vi "Dashboard Main.vi"() -> ()   [LabVIEW 2015]
uses:
  <vilib>/Utility/miscctls.llb/LVRowAndColumnTypeDef.ctl
  <vilib>/event_ctls.llb/eventvkey.ctl
  <vilib>/Rock Robotics/WPI/Dashboard/WPI_DashboardLogging Global.vi
  <vilib>/picture/3D Picture Control/Object/Create Object (name).vi
  <vilib>/Rock Robotics/Network Tables/NT Read Numeric Array.vi
  <vilib>/Rock Robotics/Network Tables/NT Write Boolean.vi
  <vilib>/Rock Robotics/Network Tables/NT Read Boolean Array.vi
  <vilib>/Rock Robotics/Network Tables/NT Read Boolean.vi
  <vilib>/Rock Robotics/Network Tables/NT Write String Array.vi
  <vilib>/Rock Robotics/Network Tables/NT Write Numeric Array.vi
  <vilib>/Utility/config.llb/Write Key (String).vi
  <vilib>/Utility/config.llb/Write Key (I32).vi
  <vilib>/Utility/config.llb/NI_LVConfig.lvlib
  <vilib>/picture/3D Picture Control/NI_3D Picture Control.lvlib
panel:
  out "NT Connected":bool
  in  "TCP":refnum<k5>
  in  "Rec Mode":enum32{"Stop", "Record", "Playback"}(radio)
  in  "Vision":u16(ring) items=["Camera Off", "USB Camera SW", "USB Camera HW", "IP Camera"]
  out "Camera IP":string
  out "Image Message":string="Timeout in Camera Communications"
  in  "Dashboard Tab":T1(tab)
  out "DD Up?":bool
  out "Intake Up?":bool
  out "Gyro Z Angle":dbl format="%#_4f"
  in  "Custom Drive?":bool=TRUE
  in  "Refresh \nRoutines":bool
  in  "Auto Routines":string(combo)
  in  "Camera Settings":T2={"Frame Rate"=30, "Compression"=30, "Size"=1} {"Frame Rate" scale=1.0..30.0; "Size" items=["640x480", "320x240", "160x120"]}
  out "MotorChart R":cluster{"Numeric":dbl, "Numeric":dbl}(graph)
  out "MotorChart L":T3(graph)
  out "MotorSliders R":cluster{"MotorSlide1":dbl, "MotorSlide2":dbl} {"MotorSlide2" scale=-1.0..1.0 scale format="%#_2e"; "MotorSlide1" scale=-1.0..1.0 scale format="%#_2e"}
  out "MotorSliders L":T4 {"MotorSlide4 2" scale=0.0..14.0 scale format="%#_2e"; "MotorSlide2" scale=-1.0..1.0 scale format="%#_2e"; "MotorSlide1" scale=-1.0..1.0 scale format="%#_2e"}
  out "Gyro Z Angle":dbl(knob) scale=0.0..360.0
  out "JS1 Z":dbl(slide) scale=-1.0..1.0 scale format="%#_2e"
  out "JS1 Graph":cluster{"X":dbl, "Y":dbl}[](graph)
  out "JS1 Buttons":T5
  out "JS2 Z":dbl(slide) scale=-1.0..1.0 scale format="%#_2e"
  out "JS2 Graph":cluster{"X":dbl, "Y":dbl}[](graph)
  out "JS2 Buttons":T5
  out "Mode":T6(ring)=enum."Auto Disabled"
  in  "DB Camera Config":bool
  out "fps":dbl format="%#.1g"
  out "Mbps":dbl format="%#.1g"
  out "Mbps 2":bool
  out "Robot Current":T7(graph)
  out "Compressor On?":bool
  out "System Current":T7(graph)
  out "Robot Position":refnum<vi>(3d-picture)
  out "IMU Angle":cluster{"X":dbl, "Y":dbl, "Z":dbl}
  out "IMU AHRS":cluster{"Pitch":dbl, "Roll":dbl, "Yaw":dbl}
  out "Right Encoder":dbl(knob) scale=0.0..256.0
  out "Right Encoder Numeric":dbl
  out "Left Encoder Numeric":dbl
  out "Left Encoder":dbl(knob) scale=0.0..256.0
  out "Tree":string(tree)
  in  "Test Slider":dbl(slide) scale=0.0..100.0 scale format="%#_3g"
  in  "On/Off":bool caption="Solenoid"
  in  "Test Name":u16(ring) items=["Select the test to run..."]
  in  "Test Tree":string(tree)
  in  "Motor":cluster{"Value":dbl, "Enable":bool} {"Value" scale=-1.0..1.0 scale format="%#_3g"}
  out "Progress":T8 {"Test Progress" scale=0.0..100.0}
  in  "Rev/Fwd":cluster{"Forward":bool, "Reverse":bool}
  in  "Test Ring":u16(ring) items=["Monochrome", "Color"]
  out "Cmd Status":string
  in  "Execute Command":bool
  in  "Command Params":string[][](table)
  in  "Command Selection":i32(listbox)
  in  "CheckList":i32(listbox)
  out "Camera Image":T9(plugin-control)
  out "Boolean":bool
  # "Left"
  # "Front"
  # "Right"
  # "Battery"
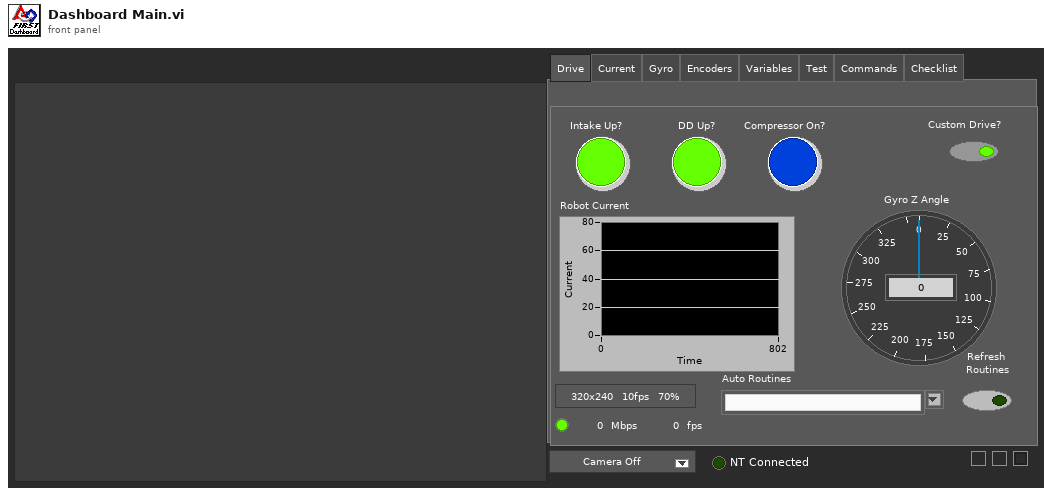
[diagram p1: front panel]
types:
  T1 = enum32{"Drive", "Current", "Gyro", "Encoders", "Variables", "Test", "Commands", "Checklist"}
  T2 = cluster{"Frame Rate":i32, "Compression":i32, "Size":u16}
  T3 = cluster{"Numeric":dbl, "Numeric":dbl, "Battery V":dbl}
  T4 = cluster{"MotorSlide1":dbl, "MotorSlide2":dbl, "MotorSlide4 2":dbl}
  T5 = cluster{bool, bool, bool, bool, bool, bool, bool, bool, bool, bool, bool, bool}
  T6 = enum8{"Tele-Op Disabled", "Tele-Op Enabled", "Auto Disabled", "Auto Enabled", "Test Disabled", "Test Enabled", "Disconnected", "No Code", "E-Stop"}
  T7 = cluster{"Numeric":dbl, "Numeric":dbl, "Numeric":dbl, "Numeric":dbl, "Numeric":dbl}
  T8 = cluster{"Test Progress":u8, "Test Progress Text":string}
  T9 = typedef "IMAQ Image.ctl" = refnum<image>
  T10 = cluster{"IDs":cluster{"RPC field ID":u16, "Unique ID":u16}, "String":string}
  T11 = enum32{"Drive", "Basic", "Custom", "Test", "Checklist", "Variables"}
  T12 = typedef "Image Type" = u32
  T13 = cluster{"Camera Image":refnum<vi>, "Dashboard Tab":refnum<vi>, "Boolean":refnum<vi>, "Vision":refnum<vi>, "Rec Mode":refnum<vi>, "Test Slider":refnum<vi>, "On/Off ":refnum<vi>, "Test Ring":refnum<vi>, "Rev/Fwd":refnum<vi>, "Test Name":refnum<vi>, "Motor":refnum<vi>, "Progress":refnum<vi>, "CheckList":refnum<vi>, "Tree":refnum<vi>, "Test Tree":refnum<vi>, "Command Params":refnum<vi>, "Command Selection":refnum<vi>, "Execute Command":refnum<vi>, "Cmd Status":refnum<vi>}
  T14 = cluster{"Match Time":dbl, "Left Master":dbl, "Left Slave":dbl, "Right Master":dbl, "Right Slave":dbl, "Battery V":dbl, "Pitch":dbl, "Roll":dbl, "Yaw":dbl, "X Angle":dbl, "Y Angle":dbl, "Z Angle":dbl, "Compressor I":dbl}
  T15 = cluster{"Error Strings":string, "Disable Counts":cluster{u16, u16}, "Rail Faults":cluster{u16, u16, u16}, "Robot IP":string, "DB Mode":u8, "Event Info":cluster{"Name":string, "Type":u8, "Number":u16, "Replay":u8}, "Camera Addr":string}
  T16 = cluster{"Storage":cluster{"Disk Free":u64, "RAM Block":u32, "RAM free":u32}, "CPU Utilization":cluster{"CPU % ISR":sgl, "CPU % Time Crit":sgl, "CPU % Timed Str":sgl, "CPU % High":sgl, "CPU % Above":sgl, "CPU % Normal":sgl, "CPU % Low":sgl}, "CAN":cluster{"% Bus Utilization":sgl, "Bus Off Cnt":u32, "TX_FIFO Full Cnt":u32, "Receive Error Cnt":u8, "Transmit Error Cnt":u8}, "HID":cluster{"HID Outputs":u32, "Rumble Low":u16, "Rumble High":u16}[]}
  T17 = cluster{"Status bits":cluster{"Test Mode":bool, "Autonomous":bool, "Enabled":bool, "Code Start":bool, "Brownout":bool, "Reserved 2":bool, "Reserved 3":bool, "E-Stop":bool}, "Code Trace":cluster{"Disabled":bool, "TeleOp":bool, "Auto":bool, "Test":bool}, "Controller Type":enum16{"unknown", "cRIO", "roboRio"}, "Code?":enum16{"unknown", "noCode", "code"}, "Battery V":dbl}
  T18 = cluster{"Control Bits":cluster{"TestMode":bool, "Autonomous":bool, "Enabled":bool, "FMS Present":bool, bool, bool, bool, "E-Stop":bool}, "Team Station ":u8, "Countdown":sgl, "Joystick Values":cluster{"Axes":dbl[], "Buttons":bool[], "POVs":i16[]}[]}
  T19 = cluster{"Axes":dbl[], "Buttons":bool[], "POVs":i16[]}[]
  T20 = cluster{"Numeric Array[0]":dbl, "Numeric Array[1]":dbl, "Numeric Array[2]":dbl, "Numeric Array[3]":dbl, "Numeric Array[4]":dbl, "Numeric Array[5]":dbl, "Numeric Array[6]":dbl, "Numeric Array[7]":dbl, "Numeric Array[8]":dbl}
  T21 = cluster{"Axes":dbl[], "Buttons":bool[], "POVs":i16[]}
  T22 = cluster{"Buttons[0]":bool, "Buttons[1]":bool, "Buttons[2]":bool, "Buttons[3]":bool, "Buttons[4]":bool, "Buttons[5]":bool, "Buttons[6]":bool, "Buttons[7]":bool, "Buttons[8]":bool, "Buttons[9]":bool, "Buttons[10]":bool, "Buttons[11]":bool}
  T23 = typedef "NI_LVConfig.lvlib/Config Data RefNum.ctl" = refnum<k1>
  T24 = cluster{"Operation":enum16{"Update", "Clear"}, "Color Box":u32}[]
  T25 = typedef "eventvkey.ctl" = enum16{"ASCII", "Enter", "Return", "Shift", "Ctrl", "Alt", "Cmd", "Opt", "Caps", "NumLock", "Clear", "Break", "Up", "Down", "Left", "Right", "Insert", "Delete", "Home", "End", "PageUp", "PageDown", "Escape", "Help", "Pause", "ScrollLock", "F1", "F2", "F3", "F4", "F5", "F6", "F7", "F8", "F9", "F10", "F11", "F12", "F13", "F14", "F15", "F16", "F17", "F18", "F19", "F20", "F21", "F22", "F23", "F24", "Play", "VolumeUp", "VolumeDown", "Mute", "Two Byte Char"}
  T26 = cluster{"Image Size":bool, "Image Type":bool, "Pixel Value":bool, "ROI Information":bool, "Zoom Factor":bool}
  T27 = enum8{"Enabled", "Disabled", "Disabled and Grayed Out"}
  T28 = cluster{"Operation":enum16{"Update", "Clear"}, "Color Box":u32}
  T29 = typedef "LVRowAndColumnTypeDef.ctl" = cluster{"Row":i32, "Column":i32}
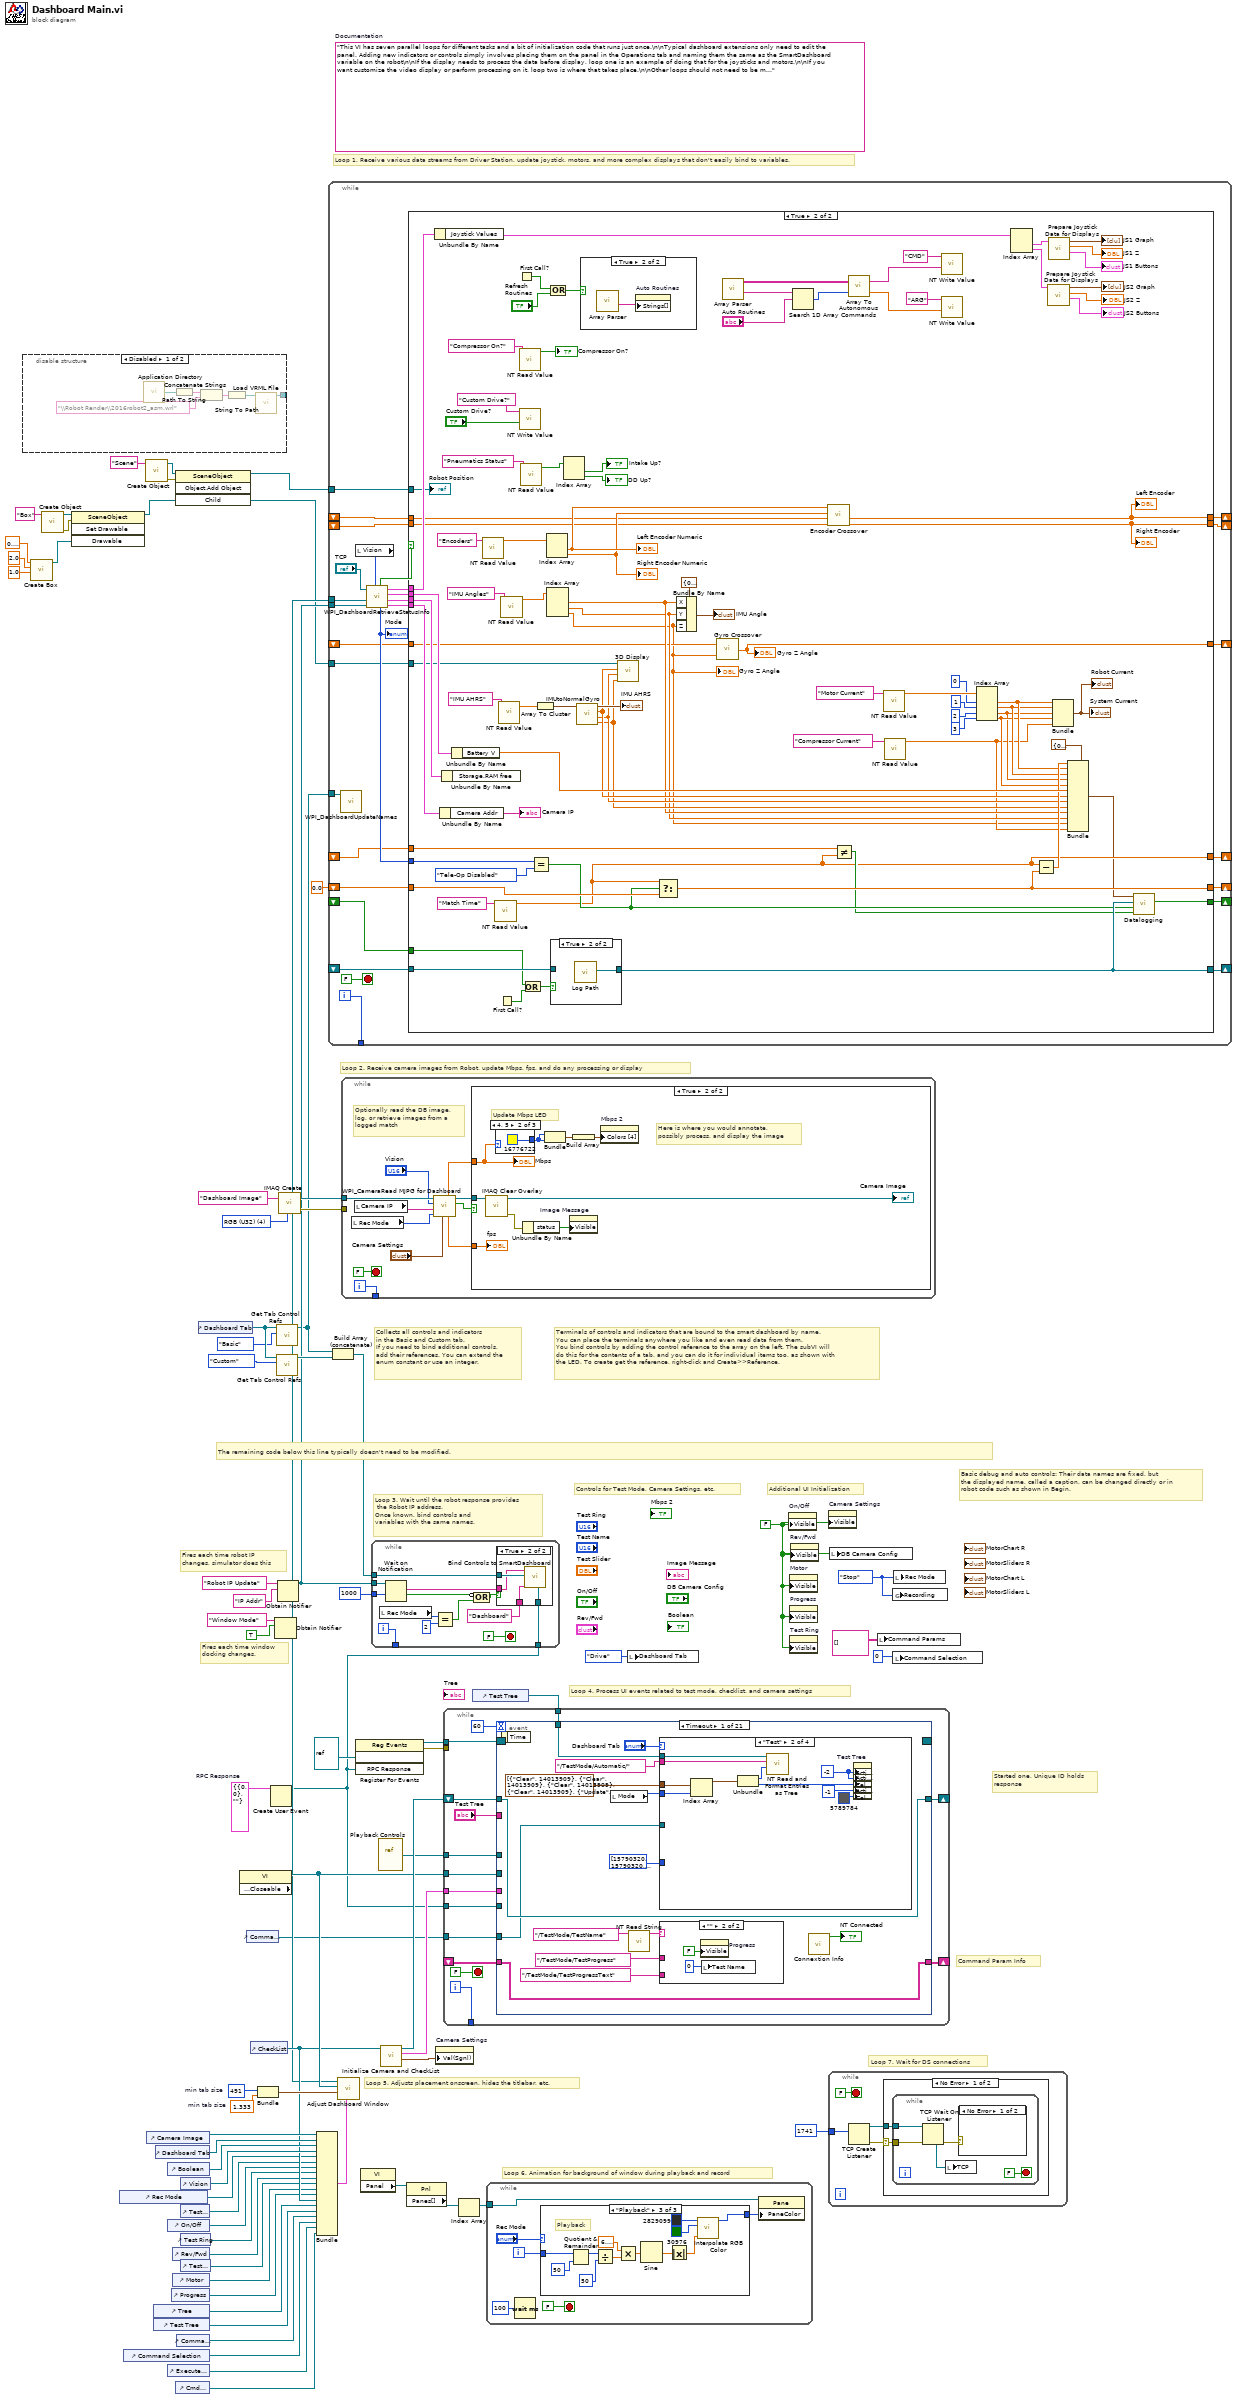
[diagram p0: block diagram]
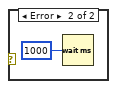
[diagram p3: hidden frame]
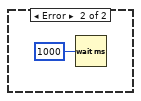
[diagram p4: hidden frame]
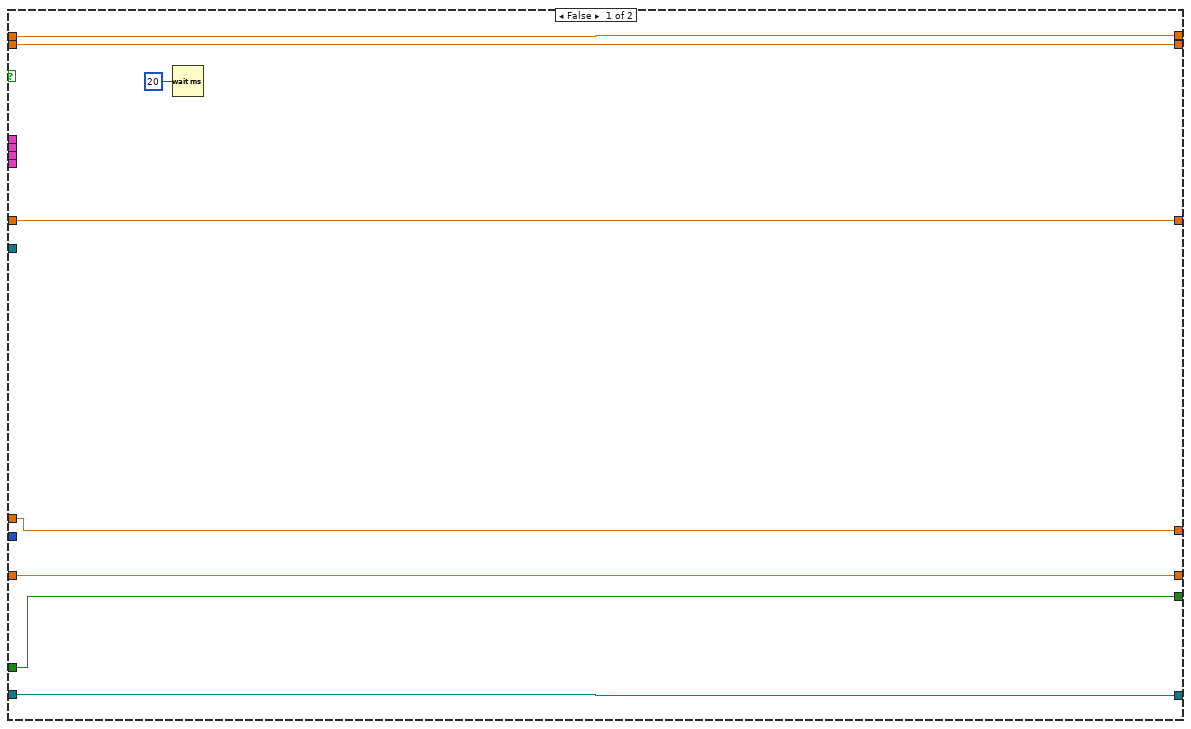
[diagram p5: hidden frame]
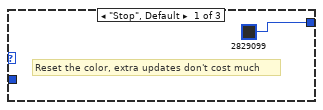
[diagram p8: hidden frame]
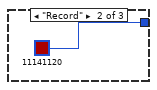
[diagram p9: hidden frame]
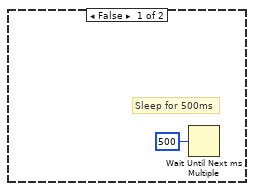
[diagram p11: hidden frame]
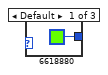
[diagram p12: hidden frame]
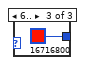
[diagram p13: hidden frame]
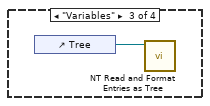
[diagram p15: hidden frame]
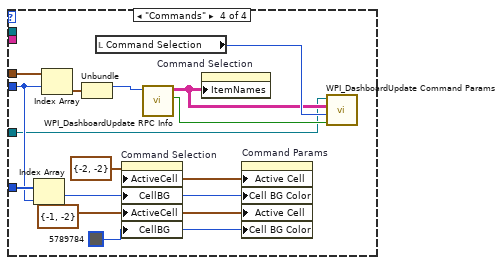
[diagram p16: hidden frame]
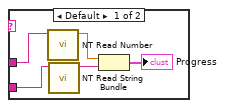
[diagram p17: hidden frame]
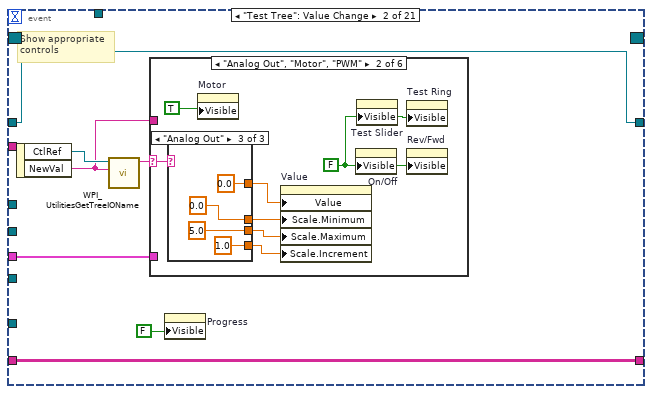
[diagram p18: hidden frame]
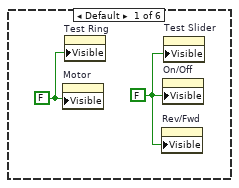
[diagram p19: hidden frame]
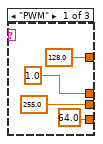
[diagram p20: hidden frame]
diagram:
  w22 = T10 {"IDs"={"RPC field ID"=0, "Unique ID"=0}, "String"=""}  # RPC Response
  w47 = 491  # min tab size
  w46 = 1.333  # min tab size
  w55 = enum32{"Stop", "Record", "Playback"}."Stop" ("Rec Mode")
  w29 = FALSE ("Visible")
  (unwired) "This VI has seven parallel loops for different tasks and a bit of initialization code that runs just once.\n\nTypical dashboard extensions only need to edit the panel. Adding new indicators or controls simply involves placing them on the panel in the Operations tab and naming them the same as the SmartDashboard variable on the robot\n\nIf the display needs to process the data before display, loop one is an example of doing that for the joysticks and motors.\n\nIf you want customize the video display or perform processing on it, loop two is where that takes place.\n\nOther loops should not need to be modified. They are pretty standard, and document the task they perform."  # Documentation
  w75 = T12 4 items=["Grayscale (U8)", "Grayscale (I16)", "Grayscale (SGL)", "Complex (CSG)", "RGB (U32)", "HSL (U32)", "RGB (U64)"] ("Image Type")
  # "Command Param Info"
  # "Started one, Unique ID holds\nresponse"
  # "Loop 7. Wait for DS connections"
  # "Basic debug and auto controls: Their data names are fixed, but\nthe displayed name, called a caption, can be changed directly or in\nrobot code such as shown in Begin."
  # "Controls for Test Mode, Camera Settings, etc."
  # "Additional UI Initialization"
  # "Loop 6. Animation for background of window during playback and record"
  # "Fires each time robot IP\nchanges, simulator does this"
  # "Fires each time window\ndocking changes."
  # "Collects all controls and indicators\nin the Basic and Custom tab.\nIf you need to bind additional controls,\nadd their references. You can extend the\nenum constant or use an integer."
  # "The remaining code below this line typically doesn't need to be modified."
  # "Loop 4. Process UI events related to test mode, checklist, and camera settings"
  # "Terminals of controls and indicators that are bound to the smart dashboard by name.\nYou can place the terminals anywhere you like and even read data from them.\nYou bind controls by adding the control reference to the array on the left. The subVI will\ndo this for the contents of a tab, and you can do it for individual items too, as shown with\nthe LED. To create get the reference, right-click and Create>>Reference."
  # "Loop 3. Wait until the robot response provides\n the Robot IP address.\nOnce known, bind controls and\nvariables with the same names."
  # "Loop 5. Adjusts placement onscreen, hides the titlebar, etc."
  # "Loop 1. Receive various data streams from Driver Station, update joystick, motors, and more complex displays that don't easily bind to variables."
  # "Loop 2. Receive camera images from Robot, update Mbps, fps, and do any processing or display"
  n1 = disable-structure shown="Disabled" {
    disable-tunnel: [w77 _] -> _
    frame Disabled {
      n2 = call <vilib>:"Application Directory.vi"() -> ("Application Directory"=w76:path)
      n3 = Path To String(path=w76) -> (string=w81:string)
      n4 = Concatenate Strings(w81, "\\Robot Render\\2016robot2_asm.wrl" ("string")) -> (w79:string)
      n5 = String To Path(string=w79) -> (path=w78:path)
      n6 = call <vilib>:"Load VRML File.vi"("Path"=w78) -> ("Scene:Read Scene File"=w77:refnum<vi>)  [unwired: 9 in, 1 out]
    }
    frame Enabled {
    }
  }
  n7 = call <vilib>:"Create Box.vi"("Length Z"=sgl 1.0, "Length Y"=sgl 2.0, "Length X"=sgl 0.2) -> ("New Box Refnum"=w9:refnum<vi>)  [unwired: 7 in, 1 out]
  n8 = call-poly <vilib>:"Create Object.vi"("Name"="Box") -> ("error out"=w8:errorcluster, "Scene:New Object"=w7:refnum<vi>)  [unwired: 9 in]
  n9 = invoke class="SceneObject" method="Set Drawable"(reference=w7, error in=w8, "Drawable"=w9) -> (reference out=w13:refnum<vi>)  [unwired: 1 in, 3 out]
  n10 = control-ref of="Rec Mode"() -> (w35:refnum<vi>)
  n11 = control-ref of="Command Selection"() -> (w21:refnum<vi>)
  n12 = call-poly <vilib>:"Create Object.vi"("Name"="Scene") -> ("error out"=w12:errorcluster, "Scene:New Object"=w11:refnum<vi>)  [unwired: 9 in]
  n13 = control-ref of="Camera Image"() -> (w50:refnum<vi>)
  n14 = control-ref of="Tree"() -> (w39:refnum<vi>)
  n15 = control-ref of="Test Tree"() -> (w38:refnum<vi>)
  n16 = control-ref of="Dashboard Tab"() -> (w49:refnum<vi>)
  n17 = control-ref of="Execute Command"() -> (w23:refnum<vi>)
  n18 = control-ref of="Boolean"() -> (w44:refnum<vi>)
  n19 = control-ref of="On/Off"() -> (w33:refnum<vi>)
  n20 = control-ref of="Progress"() -> (w30:refnum<vi>)
  n21 = control-ref of="Rev/Fwd"() -> (w31:refnum<vi>)
  n22 = control-ref of="Motor"() -> (w36:refnum<vi>)
  n23 = invoke class="SceneObject" method="Object.Add Object"(reference=w11, error in=w12, "Child"=w13) -> (reference out=w2:refnum<vi>, "Child"=w1:refnum<vi>)  [unwired: 1 in, 2 out]
  n24 = control-ref of="Cmd Status"() -> (w17:refnum<vi>)
  n25 = control-ref of="Command Params"() -> (w24:refnum<vi>)
  n26 = control-ref of="Test Slider"() -> (w34:refnum<vi>)
  n27 = control-ref of="Vision"() -> (w48:refnum<vi>)
  n28 = control-ref of="Test Ring"() -> (w32:refnum<vi>)
  n29 = control-ref of="Test Name"() -> (w37:refnum<vi>)
  n30 = control-ref of="Dashboard Tab"() -> (w53:refnum<vi>)
  n31 = property class="VI" props=["Front Panel.Closeable"]() -> (reference out=w54:refnum<vi>)  [unwired: 2 in, 2 out]
  n32 = control-ref of="Command Params"() -> (w16:refnum<vi>)
  n33 = control-ref of="CheckList"() -> (w40:refnum<vi>)
  n34 = Bundle("min tab size"=w47, "min tab size"=w46) -> (w45:cluster{"min tab size":i32, "min tab size":dbl})  [unwired: 1 in]
  n35 = Create User Event(user event datatype=w22) -> (user event=w18:refnum<user-event>)  [unwired: 1 in, 1 out]
  n36 = Obtain Notifier(name (unnamed)="Window Mode", notification data type=TRUE) -> (notifier out=w26:refnum<notifier>)  [unwired: 2 in, 2 out]
  n37 = call <vilib>:"Get Tab Control Refs.vi"("Page Index"=T11."Basic" ("Dashboard Tab"), "TabControl in"=w53) -> ("ControlsOnPage"=w27:refnum<vi>[])  [unwired: 9 in]
  n38 = call <vilib>:"Get Tab Control Refs.vi"("Page Index"=T11."Custom" ("Dashboard Tab"), "TabControl in"=w53) -> ("ControlsOnPage"=w52:refnum<vi>[])  [unwired: 9 in]
  n39 = Obtain Notifier(name (unnamed)="Robot IP Update", notification data type="IP Addr" ("name (unnamed)")) -> (notifier out=w28:refnum<notifier>)  [unwired: 2 in, 2 out]
  n40 = call "IMAQ Create"("Image Name"="Dashboard Image", "Image Type"=w75) -> ("New Image"=w73:T9, "error out"=w72:errorcluster)  [unwired: 2 in, 1 out]
  n41 = Bundle("Camera Image"=w50, "Dashboard Tab"=w49, "Boolean"=w44, "Vision"=w48, "Rec Mode"=w35, "Test Slider"=w34, "On/Off"=w33, "Test Ring"=w32, "Rev/Fwd"=w31, "Test Name"=w37, "Motor"=w36, "Progress"=w30, "CheckList"=w40, "Tree"=w39, "Test Tree"=w38, "Command Params"=w24, "Command Selection"=w21, "Execute Command"=w23, "Cmd Status"=w17) -> (w41:T13)  [unwired: 1 in]
  n42 = while {
    tunnel: [w109] -> _
    tunnel: w28 -> [w103]
    tunnel: w27 -> [w102]
    tunnel: w26 -> [w98]
    shift-right: [w96] -> _
    shift-left: _ -> [w97]
    shift-right: [w95] -> _
    shift-left: _ -> [w94]
    shift-right: [w92] -> _
    shift-left: 0.0 -> [w93]
    shift-right: [w91] -> _
    shift-left: _ -> [w90]
    tunnel: w2 -> [w89]
    shift-right: [w87] -> _
    shift-left: _ -> [w88]
    shift-right: [w85] -> _
    shift-left: _ -> [w86]
    tunnel: w1 -> [w84]
    shift-right: [w82] -> _
    shift-left: _ -> [w83]
    i -> [w109]
    stop <- FALSE stop-if-true
    n43 = call <vilib>:"WPI_DashboardUpdateNames.vi"("Controls on Tab"=w102) -> ()  [unwired: 11 in]
    n44 = local read "Vision"() -> (w100:u16)
    n45 = call <vilib>:"WPI_DashboardRetrieveStatusInfo.vi"("Vision"=w100, "Binding Refnum"=w103, "Window Mode Notifier"=w98, "TCP Cnx"="TCP") -> ("Power and Errors"=w104:T15, "Robot Metrics"=w107:T16, "Status Info"=w108:T17, "Control Info"=w105:T18, "Robot Mode"=w101:T6, "Process?"=w106:bool)  [unwired: 2 in]
    "Mode" <- w101
    n46 = case shown="True" w106 {
      tunnel: w108 -> [_ w209]
      tunnel: w107 -> [_ w208]
      tunnel: w105 -> [_ w207]
      tunnel: w104 -> [_ w206]
      tunnel: w101 -> [_ w168]
      tunnel: [w117 w178] -> w96
      tunnel: w97 -> [w117 w179]
      tunnel: [w116 w174] -> w95
      tunnel: w94 -> [w116 w173]
      tunnel: w93 -> [w115 w170]
      tunnel: [w115 w165] -> w92
      tunnel: [w114 w162] -> w91
      tunnel: w90 -> [w114 w163]
      tunnel: w89 -> [_ w161]
      tunnel: w88 -> [w113 w155]
      tunnel: [w113 w158] -> w87
      tunnel: w86 -> [w112 w154]
      tunnel: [w112 w153] -> w85
      tunnel: w84 -> [_ w128]
      tunnel: w83 -> [w111 w127]
      tunnel: [w111 w126] -> w82
      frame False {
        n47 = Wait (ms)(milliseconds to wait=u32 20) -> ()  [unwired: 1 out]
      }
      frame True {
        n48 = Unbundle By Name(w207) -> ("Joystick Values"=w205:T19)
        n49 = Unbundle By Name(w206) -> ("Camera Addr"=→"Camera IP":string)
        n50 = Unbundle By Name(w208) -> ()  [unwired: 1 out]
        n51 = Unbundle By Name(w209) -> ("Battery V"=w180:dbl)
        n52 = call-poly <vilib>:"NT Read Value.vi"("Name"="Encoders") -> ("Numeric Array"=w159:dbl[])  [unwired: 9 in, 1 out]
        n53 = call-poly <vilib>:"NT Read Value.vi"("Name"="Match Time") -> ("Numeric"=w162:dbl)  [unwired: 9 in, 1 out]
        n54 = First Call?() -> (First Call?: T/F=w172:bool)
        n55 = call-poly <vilib>:"NT Read Value.vi"("Name"="IMU AHRS") -> ("Numeric Array"=w149:dbl[])  [unwired: 9 in, 1 out]
        n56 = call-poly <vilib>:"NT Read Value.vi"("Name"="IMU Angles") -> ("Numeric Array"=w151:dbl[])  [unwired: 9 in, 1 out]
        n57 = First Call?() -> (First Call?: T/F=w177:bool)
        n58 = call-poly <vilib>:"NT Read Value.vi"("Name"="Compressor On?") -> ("Boolean"=→"Compressor On?":bool)  [unwired: 9 in, 1 out]
        n59 = call-poly <vilib>:"NT Write Value.vi"("Boolean"="Custom Drive?", "Name"="Custom Drive?") -> ()  [unwired: 9 in, 1 out]
        n60 = call-poly <vilib>:"NT Read Value.vi"("Name"="Pneumatics Status") -> ("Boolean Array"=w123:bool[])  [unwired: 9 in, 1 out]
        n61 = Or(x=w173, y=w172) -> (x .or. y?=w171:bool)
        n62 = Equal?(x=w168, y=T6."Tele-Op Disabled" ("Robot Mode")) -> (x = y?=w166:bool)
        n63 = Array To Cluster(array=w149) -> (cluster=w147:T20)
        n64 = Index Array(array=w159) -> (element #1=w157:dbl, element #2=w156:dbl)  [unwired: 2 in]
        "Left Encoder Numeric" <- w157
        "Right Encoder Numeric" <- w156
        n65 = Index Array(array=w151) -> (element #1=w138:dbl, element #2=w137:dbl, element #3=w125:dbl)  [unwired: 3 in]
        "Gyro Z Angle" <- w125
        n66 = Or(x=w177, y="Refresh \nRoutines") -> (x .or. y?=w176:bool)
        n67 = case shown="True" w171 {
          tunnel: [w210 w211] -> w178
          tunnel: w179 -> [w210 _]
          frame False {
          }
          frame True {
            n68 = call "Log Path.vi"() -> ("Log File Reference"=w211:refnum<file>)  [unwired: 11 in]
          }
        }
        n69 = Index Array(array=w123) -> (element #1=→"Intake Up?":bool, element #2=→"DD Up?":bool)  [unwired: 2 in]
        n70 = call "IMUtoNormalGyro.vi"("IMU Data"=w147) -> ("Yaw"=w142:dbl, "Roll"=w143:dbl, "Pitch"=w144:dbl, "IMU Data Out"=→"IMU AHRS":cluster{"Pitch":dbl, "Roll":dbl, "Yaw":dbl})  [unwired: 5 in]
        n71 = case shown="True" w176 {
          frame False {
          }
          frame True {
            n72 = call "Array Parser.vi"() -> ("Auto Routines"=w212:string[])  [unwired: 9 in, 2 out]
            n73 = property on="Auto Routines" class="CmbBox"("Strings[]"=w212) -> ()  [unwired: 2 in, 2 out]
          }
        }
        n74 = call "3D Display.vi"("Yaw"=w142, "Roll"=w143, "Pitch"=w144, "Object Refnum In"=w128) -> ()  [unwired: 7 in, 1 out]
        n75 = Select(t=w162, s=w166, f=w170) -> (s? t:f=w165:dbl)
        n76 = Bundle By Name(cluster=cluster{"X":dbl, "Y":dbl, "Z":dbl} {"X"=0.0, "Y"=0.0, "Z"=0.0} ("IMU Angles"), "X"=w138, "Y"=w137, "Z"=w125) -> (→"IMU Angle":cluster{"X":dbl, "Y":dbl, "Z":dbl})
        n77 = call "Gyro Crossover.vi"("Gyro Value"=w125, "Previous Value"=w127) -> ("Gyro Value"=w126:dbl)
        "Gyro Z Angle" <- w126
        n78 = call "Array Parser.vi"() -> ("Auto Routines"=w190:string[], "CSV Data"=w188:string[][][])  [unwired: 9 in, 1 out]
        n79 = Search 1D Array(1D array=w190, element="Auto Routines") -> (index of element=w189:i32)  [unwired: 1 in]
        n80 = call "Encoder Crossover.vi"("Previous Value 2"=w154, "Previous Value"=w155, "Encoder Value 2"=w156, "Encoder Value"=w157) -> ("Encoder Output 2"=w153:dbl, "Encoder Output"=w158:dbl)  [unwired: 2 in]
        "Left Encoder" <- w158
        "Right Encoder" <- w153
        n81 = Not Equal?(x=w163, y=w162) -> (x != y?=w164:bool)
        n82 = call "Array To Autonomous Commands.vi"("Which"=w189, "Input Array"=w188) -> ("Float Output Array"=w192:dbl[], "String Output Array"=w193:string[])
        n83 = call-poly <vilib>:"NT Read Value.vi"("Name"="Motor Current") -> ("Numeric Array"=w186:dbl[])  [unwired: 9 in, 1 out]
        n84 = call-poly <vilib>:"NT Read Value.vi"("Name"="Compressor Current") -> ("Numeric"=w131:dbl)  [unwired: 9 in, 1 out]
        n85 = call-poly <vilib>:"NT Write Value.vi"("String Array"=w193, "Name"="CMD") -> ()  [unwired: 9 in, 1 out]
        n86 = call-poly <vilib>:"NT Write Value.vi"("Numeric Array"=w192, "Name"="ARG") -> ()  [unwired: 9 in, 1 out]
        n87 = Index Array(array=w186, index #1=0 ("index"), index #2=1 ("index"), index #3=2 ("index"), index #4=3 ("index")) -> (element #1=w135:dbl, element #2=w134:dbl, element #3=w132:dbl, element #4=w133:dbl)
        n88 = Index Array(array=w205) -> (element #1=w204:T21, element #2=w199:T21)  [unwired: 2 in]
        n89 = Subtract(x=w162, y=w165) -> (x-y=w169:dbl)
        n90 = call "Prepare Joystick Data for Displays.vi"("Joystick Values"=w199) -> ("Buttons"=→"JS2 Buttons":T22, "Z Axis"=→"JS2 Z":dbl, "Cartesian Data"=→"JS2 Graph":cluster{"X axis":dbl, "X axis":dbl}[])  [unwired: 8 in]
        n91 = call "Prepare Joystick Data for Displays.vi"("Joystick Values"=w204) -> ("Buttons"=→"JS1 Buttons":T22, "Z Axis"=→"JS1 Z":dbl, "Cartesian Data"=→"JS1 Graph":cluster{"X axis":dbl, "X axis":dbl}[])  [unwired: 8 in]
        n92 = Bundle("Numeric"=w135, "Numeric"=w134, "Numeric"=w132, "Numeric"=w133, "Numeric"=w131) -> (→"System Current" →"Robot Current":T7)  [unwired: 1 in]
        n93 = Bundle(cluster=T14 {"Match Time"=0.0, "Left Master"=0.0, "Left Slave"=0.0, "Right Master"=0.0, "Right Slave"=0.0, "Battery V"=0.0, "Pitch"=0.0, "Roll"=0.0, "Yaw"=0.0, "X Angle"=0.0, "Y Angle"=0.0, "Z Angle"=0.0, "Compressor I"=0.0} ("Logging Data"), "Match Time"=w169, "Left Master"=w135, "Left Slave"=w134, "Right Master"=w132, "Right Slave"=w133, "Battery V"=w180, "Pitch"=w144, "Roll"=w143, "Yaw"=w142, "X Angle"=w138, "Y Angle"=w137, "Z Angle"=w125, "Compressor I"=w131) -> (w141:T14)
        n94 = call "Datalogging.vi"("Logging Data"=w141, "Log File Reference"=w178, "Match Ended?"=w166, "Second Passed?"=w164) -> ("File Closed?"=w174:bool)  [unwired: 6 in]
        "Robot Position" <- w161
      }
    }
  }
  n95 = Build Array (concatenate)(w27, w52) -> (w51:refnum<vi>[])
  n96 = call "Adjust Dashboard Window.vi"("Sizing Refnums"=w41, "Size Constraints"=w45, "VI"=w54, "WIn Mode"=w26) -> ()  [unwired: 8 in]
  n97 = while {
    tunnel: w73 -> [w221]
    tunnel: w72 -> [_]
    tunnel: [w222] -> _
    i -> [w222]
    stop <- FALSE stop-if-true
    # "Optionally read the DB image,\nlog, or retrieve images from a\nlogged match"
    n98 = local read "Rec Mode"() -> (w215:enum32{"Stop", "Record", "Playback"})
    n99 = local read "Camera IP"() -> (w213:string)
    n100 = call <vilib>:"WPI_CameraRead MJPG for Dashboard.vi"("Camera Settings"="Camera Settings", "Rec Mode"=w215, "Camera IP"=w213, "Camera Mode"="Vision", "Refnum in"=w221) -> ("Active"=w219:bool, "Refnum out"=w220:T9, "FPS"=w218:dbl, "Bandwidth (Mbps)"=w217:dbl)  [unwired: 3 in]
    n101 = case shown="True" w219 {
      tunnel: w220 -> [_ w228]
      tunnel: w217 -> [_ w227]
      tunnel: w218 -> [_ w225]
      frame False {
        # "Sleep for 500ms"
        n102 = Wait Until Next ms Multiple(millisecond multiple=u32 500) -> ()  [unwired: 1 out]
      }
      frame True {
        # "Here is where you would annotate,\npossibly process, and display the image"
        # "Update Mbps LED"
        n103 = call "IMAQ Clear Overlay"("Image"=w228) -> ("error out"=w232:errorcluster, "Image Out"=→"Camera Image":T9)  [unwired: 2 in, 7 out]
        n104 = case shown="4, 5" w227 {
          tunnel: [u32 6618880 ("Color Box") u32 16776722 ("Color Box") u32 16716800 ("Color Box")] -> w229
          frame Default {
          }
          frame 4, 5 {
          }
          frame 6.. {
          }
        }
        n105 = Unbundle By Name(w232) -> ("status"=w233:bool)
        n106 = Bundle("Color Box"=w229, "Color Box"=w229) -> (w231:cluster{"Color Box":u32, "Color Box":u32})  [unwired: 1 out]
        n107 = property on="Image Message" class="Str"("Visible"=w233) -> ()  [unwired: 2 in, 2 out]
        n108 = Build Array(w231) -> (w230:cluster{"Color Box":u32, "Color Box":u32}[])
        n109 = property on="Mbps 2" class="Bool (strict)"("Colors [4]"=w230) -> ()  [unwired: 2 in, 2 out]
        "Mbps" <- w227
        "fps" <- w225
      }
    }
  }
  n110 = register-events(refnum<vi> refnum, w18) -> (reference out=w59:refnum<event-registration>, error out=w58:errorcluster)  [unwired: 2 in]
  n111 = property class="VI"() -> ("Panel"=w62:refnum<vi>)  [unwired: 2 in, 2 out]
  n112 = while {
    tunnel: w51 -> [w249]
    tunnel: w28 -> [w247]
    tunnel: [w245] -> _
    tunnel: u32 1000 ("milliseconds to wait") -> [w244]
    tunnel: w18 -> [w237]
    i -> [w245]
    stop <- FALSE stop-if-true
    n113 = local read "Rec Mode"() -> (w240:enum32{"Stop", "Record", "Playback"})
    n114 = Wait on Notification(notifier=w247, timeout in ms (-1)=w244) -> (notification=w246:string, timed out?=w242:bool)  [unwired: 2 in, 2 out]
    n115 = Equal?(x=w240, y=u16 2 ("Rec Mode")) -> (x = y?=w241:bool)
    n116 = Compound Arithmetic op=OR(invert w242, w241) -> (w243:bool)
    n117 = case shown="True" w243 {
      tunnel: w249 -> [_ w253]
      tunnel: w246 -> [_ w252]
      tunnel: "Dashboard" -> [_ w251]
      tunnel: w237 -> [_ w250]
      frame False {
      }
      frame True {
        n118 = call <vilib>:"Bind Controls to SmartDashboard.vi"("RPC ref"=w250, "Client Name"=w251, "Bound Control Refs"=w253, "Server IP Address"=w252) -> ()  [unwired: 8 in]
      }
    }
  }
  n119 = vi-ref "Playback Controls.vi"() -> (w60:refnum<vi>)
  n120 = call "Initialize Camera and CheckList.vi"("ListBox in"=w40) -> ("Cluster"=w66:cluster{"value":i32, "value":i32, "index":i32}, "Array"=w67:cluster{string[]}[], "File Refnum"=w65:T23)  [unwired: 8 in]
  n121 = property class="Pnl"(reference=w62) -> ("Panes[]"=w63:refnum<vi>[])  [unwired: 1 in, 2 out]
  n122 = property on="Camera Settings" class="Clust (strict)"("Val(Sgnl)"=w66) -> ()  [unwired: 2 in, 2 out]
  n123 = Index Array(array=w63) -> (element=w61:refnum<vi>)  [unwired: 1 in]
  n124 = control-ref of="Test Tree"() -> (w64:refnum<vi>)
  n125 = while {
    tunnel: w67 -> [w265]
    shift-right: [w264] -> _
    shift-left: w65 -> [w263]
    tunnel: [w262] -> _
    tunnel: w64 -> [w261]
    tunnel: w60 -> [w260]
    tunnel: w59 -> [w259]
    tunnel: w58 -> [_]
    tunnel: w54 -> [w258]
    tunnel: w18 -> [w257]
    tunnel: w16 -> [w256]
    shift-right: [w255] -> _
    shift-left: _ -> [w254]
    i -> [w262]
    stop <- FALSE stop-if-true
    n126 = event shown="[0] Timeout" {
      selector: w259 -> [_ _ _ _ _ _ _ _ _ _ _ _ _ _ _ _ _ _ _ _ _]
      dyn-events: [_ _ _ _ _ _ _ _ _ _ _ _ _ _ _ _ w566 _ _ _ _] -> _
      timeout: u32 60 ("milliseconds to wait") -> [_ _ _ _ _ _ _ _ _ _ _ _ _ _ _ _ _ _ _ _ _]
      tunnel: w261 -> [w278 _ _ _ _ _ _ _ _ _ _ _ _ _ _ _ _ _ _ _ _]
      tunnel: "Test Tree" -> [_ _ _ _ _ _ _ _ _ _ _ w529 w538 w541 w546 w555 _ _ _ _ _]
      tunnel: w265 -> [_ w316 _ _ _ _ _ _ _ w491 w522 _ _ _ _ _ _ _ _ _ _]
      tunnel: [w275 w315 w419 w425 w437 w449 w457 w463 w476 w490 w515 w528 w536 w540 w545 w554 w568 w584 w586 w594 w605] -> w264
      tunnel: w263 -> [w275 w315 w419 w425 w437 w449 w457 w463 w476 w489 w515 w528 w536 w540 w545 w554 w568 w584 w586 w594 w605]
      tunnel: w260 -> [_ _ _ _ _ _ _ _ _ _ _ _ _ _ _ _ w569 _ w589 _ _]
      tunnel: w258 -> [_ _ _ _ _ _ _ _ _ _ _ _ _ _ _ _ w564 _ _ _ _]
      tunnel: w257 -> [_ _ _ _ _ _ _ _ _ _ _ _ _ _ _ _ w560 _ _ _ _]
      tunnel: w256 -> [w270 _ _ _ w435 _ _ _ _ _ _ _ _ _ _ _ _ _ _ _ _]
      tunnel: [w269 w314 w418 w424 w433 w443 w454 w462 w475 w488 w514 w527 w535 w539 w544 w553 w559 w582 w585 w590 w598] -> w255
      tunnel: w254 -> [w269 w314 w418 w424 w433 _ _ w462 w475 w488 w514 w527 w535 w539 w544 w553 w559 w582 w585 w590 w598]
      event Timeout {
        n127 = event-data() -> ()  [unwired: 1 in, 1 out]
        n128 = local read "Mode"() -> (w272:T6)
        n129 = call <vilib>:"NT Read String.vi"("Name"="/TestMode/TestName") -> ("String"=w281:string)  [unwired: 9 in, 1 out]
        n130 = case shown="\"Test\"" "Dashboard Tab" {
          tunnel: w278 -> [_ w292 _ _]
          tunnel: "/TestMode/Automatic/" ("Name Pattern") -> [_ w291 _ _]
          tunnel: T24 [{"Operation"=enum."Clear", "Color Box"=14013909}, {"Operation"=enum."Clear", "Color Box"=14013909}, {"Operation"=enum."Clear", "Color Box"=14013909}, {"Operation"=enum."Clear", "Color Box"=14013909}, {"Operation"=enum."Update", "Color Box"=14013909}, {"Operation"=enum."Update", "Color Box"=16777215}, {"Operation"=enum."Clear", "Color Box"=14013909}, {"Operation"=enum."Clear", "Color Box"=14013909}, {"Operation"=enum."Clear", "Color Box"=14013909}] -> [_ w284 _ w301]
          tunnel: w272 -> [_ w283 _ w300]
          tunnel: u32[] [15790320, 15790320, 15790320, 15790320, 16777215, 16777215, 15790320, 15790320, 15790320] -> [_ _ _ w306]
          tunnel: w270 -> [_ _ _ w294]
          frame "Gyro", Default {
          }
          frame "Test" {
            w290 = -2 ("Active Item:Row Number")
            n131 = Index Array(array=w284, index=w283) -> (element=w285:T28)
            n132 = Unbundle(w285) -> ("Operation"=w286:enum16{"Update", "Clear"}, "Color Box"=w287:u32)
            n133 = call <vilib>:"NT Read and Format Entries as Tree.vi"("Operation"=w286, "Name Pattern"=w291, "Tree Refnum"=w292) -> ()  [unwired: 7 in, 2 out]
            n134 = property on="Test Tree" class="Tree (strict)"("Active Item Row Number"=w290, "ActiveColNum"=w290, "CellBG"=w287, "Active Item Row Number"=-1 ("Active Item:Row Number"), "CellBG"=u32 5789784 ("Color Box")) -> ()  [unwired: 2 in, 2 out]
          }
          frame "Variables" {
            n135 = control-ref of="Tree"() -> (w293:refnum<vi>)
            n136 = call <vilib>:"NT Read and Format Entries as Tree.vi"("Tree Refnum"=w293) -> ()  [unwired: 9 in, 2 out]
          }
          frame "Commands" {
            w302 = u32 5789784 ("Color Box")
            w303 = T29 {"Row"=-1, "Column"=-2} ("Active Cell:Active Cell")
            w305 = T29 {"Row"=-2, "Column"=-2} ("Active Cell:Active Cell")
            n137 = Index Array(array=w306, index=w300) -> (element=w304:u32)
            n138 = Index Array(array=w301, index=w300) -> (element=w299:T28)
            n139 = Unbundle(w299) -> ("Operation"=w298:enum16{"Update", "Clear"})  [unwired: 1 out]
            n140 = local read "Command Selection"() -> (w297:i32)
            n141 = property on="Command Selection" class="MCListbox (strict)"("ActiveCell"=w305, "CellBG"=w304, "ActiveCell"=w303, "CellBG"=w302) -> ()  [unwired: 2 in, 2 out]
            n142 = call <vilib>:"WPI_DashboardUpdate RPC Info.vi"("Operation"=w298) -> ("update"=w296:bool, "commands"=w295:string[][])  [unwired: 9 in]
            n143 = property on="Command Selection" class="MCListbox (strict)"("ItemNames"=w295) -> ()  [unwired: 2 in, 2 out]
            n144 = property on="Command Params" class="Tbl (strict)"("Active Cell"=w305, "Cell BG Color"=w304, "Active Cell"=w303, "Cell BG Color"=w302) -> ()  [unwired: 2 in, 2 out]
            n145 = call <vilib>:"WPI_DashboardUpdate Command Params.vi"("Update"=w296, "NewVal"=w297, "Commands"=w295, "Param Tbl"=w294) -> ()  [unwired: 7 in, 1 out]
          }
        }
        n146 = case shown="\"\"" w281 {
          tunnel: "/TestMode/TestProgress" ("Name") -> [w308 _]
          tunnel: "/TestMode/TestProgressText" ("Name") -> [w307 _]
          frame Default {
            n147 = call <vilib>:"NT Read Number.vi"("Name"=w308) -> ("Numeric"=w309:dbl)  [unwired: 9 in, 1 out]
            n148 = call <vilib>:"NT Read String.vi"("Name"=w307) -> ("String"=w310:string)  [unwired: 9 in, 1 out]
            n149 = Bundle("Numeric"=w309, "String"=w310) -> (→"Progress":cluster{"Numeric":dbl, "String":string})  [unwired: 1 in]
          }
          frame "" {
            n150 = property on="Progress" class="Clust (strict)"("Visible"=FALSE) -> ()  [unwired: 2 in, 2 out]
            n151 = local write "Test Name"(u16 0) -> ()
          }
        }
        n152 = call <vilib>:"Connextion Info.vi"() -> ("Connected"=→"NT Connected":bool)  [unwired: 10 in, 1 out]
      }
      event "Test Tree": Value Change {
        # "Show appropriate\ncontrols"
        n153 = event-data() -> ("CtlRef"=w319:refnum<vi>, "NewVal"=w317:string)  [unwired: 1 in]
        n154 = call <vilib>:"WPI_UtilitiesGetTreeIOName.vi"("NewVal"=w317, "TreeControl in"=w319) -> ("I/O Name"=w320:string)  [unwired: 9 in]
        n155 = case shown="\"Analog Out\", \"Motor\", \"PWM\"" w320 {
          selector: w320 -> [_ w327 _ w349 w358 _]
          tunnel: w317 -> [_ _ w346 w348 _ w365]
          tunnel: w316 -> [_ _ _ _ _ w364]
          frame Default {
            w322 = FALSE ("Visible")
            w321 = FALSE ("Visible")
            n156 = property on="Motor" class="Clust (strict)"("Visible"=w321) -> ()  [unwired: 2 in, 2 out]
            n157 = property on="Test Ring" class="Ring (strict)"("Visible"=w321) -> ()  [unwired: 2 in, 2 out]
            n158 = property on="Rev/Fwd" class="Clust (strict)"("Visible"=w322) -> ()  [unwired: 2 in, 2 out]
            n159 = property on="On/Off" class="Bool (strict)"("Visible"=w322) -> ()  [unwired: 2 in, 2 out]
            n160 = property on="Test Slider" class="Slide (strict)"("Visible"=w322) -> ()  [unwired: 2 in, 2 out]
          }
          frame "Analog Out", "Motor", "PWM" {
            w328 = FALSE ("Visible")
            n161 = case shown="\"Analog Out\"" w327 {
              tunnel: [1.0 ("Value") -1.0 ("Value") 0.0 ("Value")] -> w326
              tunnel: [255.0 ("Value") 1.0 ("Value") 5.0 ("Value")] -> w325
              tunnel: [128.0 ("Value") 0.0 ("Value") 0.0 ("Value")] -> w324
              tunnel: [64.0 ("Value") 0.5 ("Value") 1.0 ("Value")] -> w323
              frame "PWM" {
              }
              frame "Motor", Default {
              }
              frame "Analog Out" {
              }
            }
            n162 = property on="Motor" class="Clust (strict)"("Visible"=TRUE) -> ()  [unwired: 2 in, 2 out]
            n163 = property on="Value" class="Slide (strict)"("Value"=w324, "Scale.Minimum"=w326, "Scale.Maximum"=w325, "Scale.Increment"=w323) -> ()  [unwired: 2 in, 2 out]
            n164 = property on="On/Off" class="Bool (strict)"("Visible"=w328) -> ()  [unwired: 2 in, 2 out]
            n165 = property on="Test Slider" class="Slide (strict)"("Visible"=w328) -> ()  [unwired: 2 in, 2 out]
            n166 = property on="Test Ring" class="Ring (strict)"("Visible"=w328) -> ()  [unwired: 2 in, 2 out]
            n167 = property on="Rev/Fwd" class="Clust (strict)"("Visible"=w328) -> ()  [unwired: 2 in, 2 out]
          }
          frame "Servo" {
            w344 = FALSE ("Visible")
            n168 = call <vilib>:"NT Read Number.vi"("Name"=w346) -> ("Numeric"=w345:dbl)  [unwired: 9 in, 1 out]
            n169 = property on="Test Slider" class="Slide (strict)"("Visible"=TRUE, "Scale.Maximum"=170.0 ("Scale.Range:Maximum")) -> ()  [unwired: 2 in, 2 out]
            n170 = local write "Test Slider"(w345) -> ()
            n171 = property on="Motor" class="Clust (strict)"("Visible"=w344) -> ()  [unwired: 2 in, 2 out]
            n172 = property on="Rev/Fwd" class="Clust (strict)"("Visible"=w344) -> ()  [unwired: 2 in, 2 out]
            n173 = property on="On/Off" class="Bool (strict)"("Visible"=w344) -> ()  [unwired: 2 in, 2 out]
            n174 = property on="Test Ring" class="Ring (strict)"("Visible"=w344) -> ()  [unwired: 2 in, 2 out]
          }
          frame "Relay", "Solenoid" {
            w347 = FALSE ("Visible")
            n175 = property on="Motor" class="Clust (strict)"("Visible"=w347) -> ()  [unwired: 2 in, 2 out]
            n176 = property on="Test Slider" class="Slide (strict)"("Visible"=w347) -> ()  [unwired: 2 in, 2 out]
            n177 = Search and Replace String(input string=w348, search string="/Value  **", replace string="/Direction") -> (result string=w354:string)  [unwired: 5 in, 3 out]
            n178 = property on="Test Ring" class="Ring (strict)"("Visible"=w347) -> ()  [unwired: 2 in, 2 out]
            n179 = call <vilib>:"NT Read String.vi"("Name"=w354) -> ("String"=w352:string)  [unwired: 9 in, 1 out]
            n180 = Equal?(x="Both directions", y=w352) -> (x = y?=w350:bool)
            n181 = Not(x=w350) -> (.not. x?=w351:bool)
            n182 = property on="Rev/Fwd" class="Clust (strict)"("Visible"=w350) -> ()  [unwired: 2 in, 2 out]
            n183 = property on="On/Off" class="Bool (strict)"("Visible"=w351, "Caption.Text"=w349) -> ()  [unwired: 2 in, 2 out]
          }
          frame "Compressor", "Digital Out" {
            w357 = FALSE ("Visible")
            # "Get direction and finish"
            n184 = property on="Motor" class="Clust (strict)"("Visible"=w357) -> ()  [unwired: 2 in, 2 out]
            n185 = property on="Test Slider" class="Slide (strict)"("Visible"=w357) -> ()  [unwired: 2 in, 2 out]
            n186 = property on="Test Ring" class="Ring (strict)"("Visible"=w357) -> ()  [unwired: 2 in, 2 out]
            n187 = property on="On/Off" class="Bool (strict)"("Visible"=TRUE, "Caption.Text"=w358) -> ()  [unwired: 2 in, 2 out]
            n188 = property on="Rev/Fwd" class="Clust (strict)"("Visible"=FALSE) -> ()  [unwired: 2 in, 2 out]
          }
          frame "Camera" {
            n189 = call <vilib>:"Get Last Path Segment.vi"("String in"=w365) -> ("String out"=w366:string)  [unwired: 10 in]
            n190 = property on="On/Off" class="Bool (strict)"("Visible"=FALSE) -> ()  [unwired: 2 in, 2 out]
            n191 = property on="Motor" class="Clust (strict)"("Visible"=FALSE) -> ()  [unwired: 2 in, 2 out]
            n192 = property on="Rev/Fwd" class="Clust (strict)"("Visible"=FALSE) -> ()  [unwired: 2 in, 2 out]
            n193 = case shown="\"White Balance  **\"" w366 {
              tunnel: w365 -> [w372 w381 w390 w399 w408 _ w414]
              tunnel: w364 -> [w370 w378 w387 w396 w405 _ _]
              frame "Size  **" {
                n194 = Index Array(array=w370) -> (element=w369:cluster{string[]})  [unwired: 1 in]
                n195 = call <vilib>:"NT Read String.vi"("Name"=w372) -> ("String"=w371:string)  [unwired: 9 in, 1 out]
                n196 = Unbundle(w369) -> (w367:string[])
                n197 = Match First String(2:w367, 3:w371) -> (0:w368:i32)  [unwired: 1 out]
                n198 = property on="Test Ring" class="Ring (strict)"("Value"=w368, "Strings []"=w367) -> ()  [unwired: 2 in, 2 out]
                n199 = property on="Test Ring" class="Ring (strict)"("Visible"=TRUE) -> ()  [unwired: 2 in, 2 out]
                n200 = property on="Test Slider" class="Slide (strict)"("Visible"=FALSE) -> ()  [unwired: 2 in, 2 out]
              }
              frame "White Balance  **" {
                n201 = Index Array(array=w378, index=1) -> (element=w379:cluster{string[]})
                n202 = call <vilib>:"NT Read String.vi"("Name"=w381) -> ("String"=w380:string)  [unwired: 9 in, 1 out]
                n203 = Unbundle(w379) -> (w376:string[])
                n204 = Match First String(2:w376, 3:w380) -> (0:w375:i32)  [unwired: 1 out]
                n205 = property on="Test Ring" class="Ring (strict)"("Value"=w375, "Strings []"=w376) -> ()  [unwired: 2 in, 2 out]
                n206 = property on="Test Ring" class="Ring (strict)"("Visible"=TRUE) -> ()  [unwired: 2 in, 2 out]
                n207 = property on="Test Slider" class="Slide (strict)"("Visible"=FALSE) -> ()  [unwired: 2 in, 2 out]
              }
              frame "Exposure  **" {
                n208 = Index Array(array=w387, index=2) -> (element=w388:cluster{string[]})
                n209 = call <vilib>:"NT Read String.vi"("Name"=w390) -> ("String"=w389:string)  [unwired: 9 in, 1 out]
                n210 = Unbundle(w388) -> (w384:string[])
                n211 = Match First String(2:w384, 3:w389) -> (0:w385:i32)  [unwired: 1 out]
                n212 = property on="Test Ring" class="Ring (strict)"("Value"=w385, "Strings []"=w384) -> ()  [unwired: 2 in, 2 out]
                n213 = property on="Test Ring" class="Ring (strict)"("Visible"=TRUE) -> ()  [unwired: 2 in, 2 out]
                n214 = property on="Test Slider" class="Slide (strict)"("Visible"=FALSE) -> ()  [unwired: 2 in, 2 out]
              }
              frame "Exposure Priority  **" {
                n215 = Index Array(array=w396, index=3) -> (element=w397:cluster{string[]})
                n216 = call <vilib>:"NT Read String.vi"("Name"=w399) -> ("String"=w398:string)  [unwired: 9 in, 1 out]
                n217 = Unbundle(w397) -> (w393:string[])
                n218 = Match First String(2:w393, 3:w398) -> (0:w394:i32)  [unwired: 1 out]
                n219 = property on="Test Ring" class="Ring (strict)"("Value"=w394, "Strings []"=w393) -> ()  [unwired: 2 in, 2 out]
                n220 = property on="Test Ring" class="Ring (strict)"("Visible"=TRUE) -> ()  [unwired: 2 in, 2 out]
                n221 = property on="Test Slider" class="Slide (strict)"("Visible"=FALSE) -> ()  [unwired: 2 in, 2 out]
              }
              frame "Color Enable  **" {
                n222 = Index Array(array=w405, index=4) -> (element=w406:cluster{string[]})
                n223 = call <vilib>:"NT Read String.vi"("Name"=w408) -> ("String"=w407:string)  [unwired: 9 in, 1 out]
                n224 = Unbundle(w406) -> (w402:string[])
                n225 = Match First String(2:w402, 3:w407) -> (0:w403:i32)  [unwired: 1 out]
                n226 = property on="Test Ring" class="Ring (strict)"("Value"=w403, "Strings []"=w402) -> ()  [unwired: 2 in, 2 out]
                n227 = property on="Test Ring" class="Ring (strict)"("Visible"=TRUE) -> ()  [unwired: 2 in, 2 out]
                n228 = property on="Test Slider" class="Slide (strict)"("Visible"=FALSE) -> ()  [unwired: 2 in, 2 out]
              }
              frame Default {
                n229 = property on="Test Ring" class="Ring (strict)"("Visible"=FALSE) -> ()  [unwired: 2 in, 2 out]
                n230 = property on="Test Slider" class="Slide (strict)"("Visible"=FALSE) -> ()  [unwired: 2 in, 2 out]
              }
              frame "Brightness  **", "Color Level  **", "Compression  **", "FPS  **", "Sharpness  **" {
                n231 = call <vilib>:"NT Read Number.vi"("Name"=w414) -> ("Numeric"=w413:dbl)  [unwired: 9 in, 1 out]
                n232 = local write "Test Slider"(w413) -> ()
                n233 = property on="Test Slider" class="Slide (strict)"("Visible"=TRUE, "Scale.Maximum"=100.0 ("Scale.Range:Maximum")) -> ()  [unwired: 2 in, 2 out]
                n234 = property on="Test Ring" class="Ring (strict)"("Visible"=FALSE) -> ()  [unwired: 2 in, 2 out]
              }
            }
          }
        }
        n235 = property on="Progress" class="Clust (strict)"("Visible"=FALSE) -> ()  [unwired: 2 in, 2 out]
      }
      event "Test Name": Mouse Enter {
        # "Populate the ring with the list of tests"
        n236 = event-data() -> ()  [unwired: 1 in, 1 out]
        n237 = call <vilib>:"NT Read String Array.vi"("Name"="/TestMode/TestList") -> ("String Array"=w423:string[])  [unwired: 9 in, 1 out]
        n238 = Build Array (concatenate)("Select the test to run...", w423) -> (w422:string[])
        n239 = property on="Test Name" class="Ring (strict)"("Strings []"=w422) -> ()  [unwired: 2 in, 2 out]
      }
      event "Test Name": Value Change {
        w426 = FALSE ("Visible")
        # "Tell the robot the test name to run"
        n240 = event-data() -> ("NewVal"=w430:u16)  [unwired: 1 in]
        n241 = property on="Test Name" class="Ring (strict)"() -> ("Strings []"=w431:string[])  [unwired: 2 in, 2 out]
        n242 = local write "Progress"(T8 {"Test Progress"=0, "Test Progress Text"=""} ("Progress")) -> ()
        n243 = Index Array(array=w431, index=w430) -> (element=w429:string)
        n244 = call <vilib>:"NT Write String.vi"("String"=w429, "Name"="/TestMode/TestName") -> ()  [unwired: 9 in, 1 out]
        n245 = property on="Progress" class="Clust (strict)"("Visible"=TRUE) -> ()  [unwired: 2 in, 2 out]
        n246 = property on="Motor" class="Clust (strict)"("Visible"=w426) -> ()  [unwired: 2 in, 2 out]
        n247 = property on="Test Slider" class="Slide (strict)"("Visible"=w426) -> ()  [unwired: 2 in, 2 out]
        n248 = property on="On/Off" class="Bool (strict)"("Visible"=w426) -> ()  [unwired: 2 in, 2 out]
        n249 = property on="Rev/Fwd" class="Clust (strict)"("Visible"=w426) -> ()  [unwired: 2 in, 2 out]
        n250 = property on="Test Ring" class="Ring (strict)"("Visible"=w426) -> ()  [unwired: 2 in, 2 out]
      }
      event "Command Selection": Value Change {
        # "Get the params and show in table"
        n251 = event-data() -> ("NewVal"=w436:i32)  [unwired: 1 in]
        n252 = property on="Command Selection" class="MCListbox (strict)"() -> ("ItemNames"=w434:string[][])  [unwired: 2 in, 2 out]
        n253 = call <vilib>:"WPI_DashboardUpdate Command Params.vi"("NewVal"=w436, "Commands"=w434, "Param Tbl"=w435) -> ()  [unwired: 8 in, 1 out]
      }
      event "Execute Command": Value Change {
        # "Started one, Unique ID holds\nresponse"
        n254 = event-data() -> ()  [unwired: 1 in, 1 out]
        n255 = property on="Command Selection" class="MCListbox (strict)"() -> ("ItemNames"=w448:string[][])  [unwired: 2 in, 2 out]
        n256 = Index Array(array=w448, index (row)="Command Selection", index (col)=0) -> (element=w446:string)
        n257 = call <vilib>:"Invoke Commands.vi"("Command Params"="Command Params", "Function Name"=w446) -> ("Params"=w442:u8, "Started"=w441:bool)  [unwired: 7 in, 1 out]
        n258 = Array Subset(array="Command Params", length (row)=w442) -> (w443:string[][])  [unwired: 3 in]
        n259 = Select(t="Executing" ("Cmd Status"), s=w441, f="" ("Cmd Status")) -> (s? t:f=→"Cmd Status":string)
      }
      event "Command Selection": Double Click {
        n260 = event-data() -> ("Row"=w458:i32)  [unwired: 1 in]
        n261 = property on="Command Selection" class="MCListbox (strict)"() -> ("ItemNames"=w461:string[][])  [unwired: 2 in, 2 out]
        n262 = local read "Command Params"() -> (w456:string[][])
        n263 = Index Array(array=w461, index (row)=w458, index (col)=0) -> (element=w459:string)
        n264 = call <vilib>:"Invoke Commands.vi"("Command Params"=w456, "Function Name"=w459) -> ("Params"=w455:u8, "Started"=w450:bool)  [unwired: 7 in, 1 out]
        n265 = Array Subset(array=w456, length (row)=w455) -> (w454:string[][])  [unwired: 3 in]
        n266 = Select(t="Executing" ("Cmd Status"), s=w450, f="" ("Cmd Status")) -> (s? t:f=w451:string)
        n267 = local write "Cmd Status"(w451) -> ()
      }
      event "CheckList": Double Click {
        # "Shift clears all"
        # "Update symbols on the listbox"
        n268 = event-data() -> ("PlatMods.Shift"=w464:bool, "Row"=w466:i32)  [unwired: 1 in]
        n269 = case shown="True" w464 {
          tunnel: w466 -> [w470 _]
          tunnel: 1 -> [w469 _]
          frame False {
            n270 = property on="CheckList" class="LstBox (strict)"() -> ("Item Symbols"=w468:i32[])  [unwired: 2 in, 2 out]
            n271 = Replace Array Subset(array=w468, new element=w469, index=w470) -> (w467:i32[])
            n272 = property on="CheckList" class="LstBox (strict)"("Item Symbols"=w467) -> ()  [unwired: 2 in, 2 out]
          }
          frame True {
            w471 = 0 ("Top Row")
            n273 = property on="CheckList" class="LstBox (strict)"() -> ("Number of Rows"=w473:u32)  [unwired: 2 in, 2 out]
            n274 = Initialize Array(0, w473) -> (w472:i32[])
            n275 = property on="CheckList" class="LstBox (strict)"("Top Row"=w471, "Value"=w471, "Item Symbols"=w472) -> ()  [unwired: 2 in, 2 out]
          }
        }
      }
      event "CheckList": Key Down {
        # "Update symbols on the listbox\nLeft and right keys check and uncheck"
        n276 = event-data() -> ("VKey"=w478:T25)  [unwired: 1 in]
        n277 = case shown="\"Left\", \"Right\"" w478 {
          selector: w478 -> [w483 _]
          tunnel: eventvkey."Left" ("VKey") -> [w481 _]
          frame "Left", "Right" {
            n278 = Equal?(x=w481, y=w483) -> (x = y?=w482:bool)
            n279 = Select(t=0, s=w482, f=1) -> (s? t:f=w484:i32)
            n280 = property on="CheckList" class="LstBox (strict)"() -> ("Item Symbols"=w487:i32[])  [unwired: 2 in, 2 out]
            n281 = Replace Array Subset(array=w487, new element=w484, index="CheckList") -> (w486:i32[])
            n282 = property on="CheckList" class="LstBox (strict)"("Item Symbols"=w486) -> ()  [unwired: 2 in, 2 out]
          }
          frame Default {
          }
        }
      }
      event "DB Camera Config": Value Change {
        # "Show or hide the cluster of controls, store in ini file"
        n283 = event-data() -> ("NewVal"=w492:bool)  [unwired: 1 in]
        n284 = case shown="False" w492 {
          tunnel: w491 -> [w501 _]
          tunnel: [w494 w512] -> w490
          tunnel: w489 -> [w493 w512]
          frame False {
            w508 = "Camera"
            w511 = FALSE ("Visible")
            n285 = local read "Camera Settings"() -> (w500:T2)
            n286 = Index Array(array=w501) -> (element=w504:cluster{string[]})  [unwired: 1 in]
            n287 = Unbundle(w500) -> ("Frame Rate"=w499:i32, "Compression"=w498:i32, "Size"=w502:u16)
            n288 = Unbundle(w504) -> (w503:string[])
            n289 = Index Array(array=w503, index=w502) -> (element=w497:string)
            n290 = call-poly <vilib>:"Write Key.vi"("section"=w508, "value"=w497, "key"="Size", "refnum"=w493) -> ("refnum out"=w510:T23)  [unwired: 2 in, 5 out]
            n291 = call-poly <vilib>:"Write Key.vi"("section"=w508, "value"=w499, "key"="FrameRate", "refnum"=w510) -> ("refnum out"=w509:T23)  [unwired: 1 in, 6 out]
            n292 = property on="Camera Settings" class="Clust (strict)"("Visible"=w511) -> ()  [unwired: 2 in, 2 out]
            n293 = local write "DB Camera Config"(w511) -> ()
            n294 = call-poly <vilib>:"Write Key.vi"("section"=w508, "value"=w498, "key"="Compression", "refnum"=w509) -> ("refnum out"=w495:T23)  [unwired: 1 in, 6 out]
            n295 = call <vilib>:"Close Config Data.vi"("refnum"=w495) -> ("file path"=w496:path)  [unwired: 2 in, 8 out]
            n296 = call <vilib>:"Open Config Data.vi"("configuration file path"=w496) -> ("refnum"=w494:T23)  [unwired: 8 in, 2 out]
          }
          frame True {
            n297 = property on="Camera Settings" class="Clust (strict)"("Visible"=TRUE) -> ()  [unwired: 2 in, 2 out]
          }
        }
      }
      event "Camera Settings": Value Change {
        # "Update summary string when any elements of DB camera change"
        n298 = event-data() -> ("NewVal"=w526:T2)  [unwired: 1 in]
        n299 = Index Array(array=w522) -> (element=w521:cluster{string[]})  [unwired: 1 in]
        n300 = Unbundle(w526) -> ("Frame Rate"=w517:i32, "Compression"=w516:i32, "Size"=w519:u16)
        n301 = Unbundle(w521) -> (w520:string[])
        n302 = Index Array(array=w520, index=w519) -> (element=w518:string)
        n303 = Format Into String(format string="%s   %dfps   %d%%", w518, w517, w516) -> (resulting string=w523:string)  [unwired: 2 in, 1 out]
        n304 = Build Array(w523) -> (w524:string[])
        n305 = property on="DB Camera Config" class="Bool (strict)"("Strings [4]"=w524) -> ()  [unwired: 2 in, 2 out]
      }
      event "Motor.Enable": Value Change {
        # "When the test mode otor enable helper is set, update that\ntree row item's value"
        n306 = event-data() -> ("NewVal"=w533:bool)  [unwired: 1 in]
        n307 = Unbundle("Motor") -> ("Value"=w532:dbl)  [unwired: 1 out]
        n308 = Select(t=w532, s=w533, f=0.0) -> (s? t:f=w530:dbl)
        n309 = call <vilib>:"NT Write Number.vi"("Numeric"=w530, "Name"=w529) -> ()  [unwired: 9 in, 1 out]
      }
      event "Test Slider": Value Change {
        # "When the test mode slider helper is set, update that\ntree row item's value"
        n310 = event-data() -> ("NewVal"=w537:dbl)  [unwired: 1 in]
        n311 = call <vilib>:"NT Write Number.vi"("Numeric"=w537, "Name"=w538) -> ()  [unwired: 9 in, 1 out]
      }
      event "On/Off": Value Change {
        # "When the test mode on/off helper value is set, update that\ntree row item's value"
        n312 = event-data() -> ("NewVal"=w543:bool)  [unwired: 1 in]
        n313 = Boolean To (0,1)(Boolean=w543) -> (0, 1=w542:i16)
        n314 = call <vilib>:"NT Write Number.vi"("Numeric"=w542, "Name"=w541) -> ()  [unwired: 9 in, 1 out]
      }
      event "Rev/Fwd": Value Change {
        # "When the test mode helper value for relays is set, update that\ntree row item's value"
        n315 = event-data() -> ("NewVal.Forward"=w552:bool, "NewVal.Reverse"=w551:bool)  [unwired: 1 in]
        n316 = Boolean To (0,1)(Boolean=w552) -> (0, 1=w548:i16)
        n317 = Boolean To (0,1)(Boolean=w551) -> (0, 1=w550:i16)
        n318 = Negate(x=w550) -> (-x=w549:i16)
        n319 = Add(x=w548, y=w549) -> (x+y=w547:i16)
        n320 = call <vilib>:"NT Write Number.vi"("Numeric"=w547, "Name"=w546) -> ()  [unwired: 9 in, 1 out]
      }
      event "Test Ring": Value Change {
        # "When a test mode helper value is selected from the ring,\nset the tree item's variable to the string value"
        n321 = event-data() -> ("NewVal"=w557:u16)  [unwired: 1 in]
        n322 = property on="Test Ring" class="Ring (strict)"() -> ("Strings []"=w558:string[])  [unwired: 2 in, 2 out]
        n323 = Index Array(array=w558, index=w557) -> (element=w556:string)
        n324 = call <vilib>:"NT Write String.vi"("String"=w556, "Name"=w555) -> ()  [unwired: 9 in, 1 out]
      }
      event "Rec Mode": Value Change {
        # "Update globals for recording mode and path to read log from.\nClear when logging and let NetworkTables set path for vision to\nuse."
        n325 = event-data() -> ("NewVal"=w570:enum32{"Stop", "Record", "Playback"})  [unwired: 1 in]
        n326 = global write "WPI_DashboardLogging Global.vi" "Logging Filename"(path "") -> ()
        n327 = global write "WPI_DashboardLogging Global.vi" "Recording"(w570) -> ()
        n328 = case shown="\"Playback\"" w570 {
          tunnel: w569 -> [_ w572 w581]
          tunnel: [_ _ w580] -> w566
          tunnel: [_ _ w579] -> _
          tunnel: w564 -> [_ _ w577]
          tunnel: cluster{i32, i32} {-250, 170} -> [_ _ w576]
          tunnel: [_ _ T26 {"Image Size"=TRUE, "Image Type"=TRUE, "Pixel Value"=TRUE, "ROI Information"=TRUE, "Zoom Factor"=FALSE} ("Image Information Shown:All Elements")] -> w562
          tunnel: [_ _ TRUE ("Zoom Factor")] -> w561
          tunnel: w560 -> [_ _ w573]
          frame Default {
          }
          frame "Stop", "Record" {
            # "Place Window too"
            n329 = invoke class="VI" method="FP.Close"(reference=w572) -> (reference out=w571:refnum<vi>)  [unwired: 2 in, 2 out]
            n330 = invoke class="VI" method="Abort VI"(reference=w571) -> ()  [unwired: 2 in, 3 out]
          }
          frame "Playback" {
            n331 = call "Open Playback Panel.vi"("Offset"=w576, "DB VI Ref"=w577, "Playback in"=w581) -> ("Playback out"=w578:refnum<vi>)  [unwired: 8 in]
            n332 = register-events(w578, w573) -> (reference out=w580:refnum<event-registration>, error out=w579:errorcluster)  [unwired: 2 in]
          }
        }
        n333 = property on="Camera Image" class="ImageControl"("Image Information Shown"=w562, "Image Information Visible"=w561) -> ()  [unwired: 2 in, 2 out]
        n334 = call <vilib>:"WPI_DashboardNT Log FieldName Cache.vi"("Operation"=enum16{"Lookup/Add", "Index", "Clear"}."Clear") -> ()  [unwired: 8 in, 3 out]
      }
      event Panel Close {
        w583 = enum32{"Stop", "Record", "Playback"}."Stop" ("Rec Mode")
        # "Playback window has been closed, abort"
        n335 = event-data() -> ()  [unwired: 1 in, 4 out]
        n336 = local write "Rec Mode"(w583) -> ()
        n337 = global write "WPI_DashboardLogging Global.vi" "Recording"(w583) -> ()
      }
      event Panel Close {
        # "Abort playback window and ourself"
        n338 = event-data() -> ()  [unwired: 1 in, 4 out]
        n339 = invoke class="VI" method="FP.Close"(reference=w589) -> (reference out=w588:refnum<vi>)  [unwired: 2 in, 2 out]
        n340 = invoke class="VI" method="Abort VI"(reference=w588) -> (error out=w587:errorcluster)  [unwired: 2 in, 2 out]
        n341 = invoke class="VI" method="Abort VI"(error in=w587) -> ()  [unwired: 2 in, 3 out]
      }
      event User Event {
        n342 = event-data() -> ("IDs"=w597:cluster{"RPC field ID":u16, "Unique ID":u16}, "String"=w596:string)  [unwired: 1 in]
        n343 = Bundle("IDs"=w597, "String"=w596) -> (w595:T10)  [unwired: 1 in]
        n344 = call <vilib>:"Retrieve RPC Response.vi"("RPC Response"=w595) -> ("Output"=w592:string[][])  [unwired: 10 in]
        n345 = Build Array (concatenate)(w590, w592) -> (w591:string[][])
        n346 = local write "Command Params"(w591) -> ()
        n347 = local write "Cmd Status"("" ("Cmd Status")) -> ()
      }
      event "Vision": Value Change {
        # "Enable/Disable Compression slider.\nHW USB is hard-coded into the camera"
        n348 = event-data() -> ("NewVal"=w604:u16)  [unwired: 1 in]
        n349 = Equal?(x=w604, y=u32 2 ("milliseconds to wait")) -> (x = y?=w602:bool)
        n350 = Select(t=T27."Disabled and Grayed Out" ("Disabled"), s=w602, f=T27."Enabled" ("Disabled")) -> (s? t:f=w599:T27)
        n351 = property on="Compression" class="Slide (strict)"("DisabledEnum"=w599) -> ()  [unwired: 2 in, 2 out]
      }
    }
  }
  n352 = while {
    tunnel: w61 -> [w607]
    i -> [w610]
    stop <- FALSE stop-if-true
    n353 = Wait (ms)(milliseconds to wait=u32 100) -> ()  [unwired: 1 out]
    n354 = case shown="\"Playback\"" "Rec Mode" {
      tunnel: w610 -> [_ _ w625]
      tunnel: [u32 2829099 ("Base Color") u32 11141120 ("Target Color") w614] -> w606
      frame "Stop", Default {
        # "Reset the color, extra updates don't cost much"
      }
      frame "Record" {
      }
      frame "Playback" {
        # "Playback"
        n355 = Quotient & Remainder(x=w625, y=u32 50 ("milliseconds to wait")) -> (x-y*floor(x/y)=w621:u32)  [unwired: 1 out]
        n356 = Divide(x=w621, y=u32 50 ("milliseconds to wait")) -> (x/y=w618:dbl)
        n357 = Multiply(x=6.283185307179586, y=w618) -> (x*y=w623:dbl)
        n358 = Sine(x=w623) -> (sin(x)=w622:dbl)
        n359 = Absolute Value(x=w622) -> (abs(x)=w615:dbl)
        n360 = call "Interpolate RGB Color.vi"("Proportion"=w615, "Target Color"=u32 30976, "Base Color"=u32 2829099) -> ("Result Color"=w614:u32)  [unwired: 8 in]
      }
    }
    n361 = property class="Pane"(reference=w607, "PaneColor"=w606) -> ()  [unwired: 1 in, 2 out]
  }
  n362 = local write "Dashboard Tab"(T1."Drive" ("Dashboard Tab")) -> ()
  n363 = property on="On/Off" class="Bool (strict)"("Visible"=w29) -> ()  [unwired: 2 in, 2 out]
  n364 = property on="Motor" class="Clust (strict)"("Visible"=w29) -> ()  [unwired: 2 in, 2 out]
  n365 = property on="Progress" class="Clust (strict)"("Visible"=w29) -> ()  [unwired: 2 in, 2 out]
  n366 = property on="Test Ring" class="Ring (strict)"("Visible"=w29) -> ()  [unwired: 2 in, 2 out]
  n367 = property on="Rev/Fwd" class="Clust (strict)"("Visible"=w29) -> ()  [unwired: 2 in, 2 out]
  n368 = property on="Camera Settings" class="Clust (strict)"("Visible"=w29) -> ()  [unwired: 2 in, 2 out]
  n369 = while {
    tunnel: u16 1741 ("timeout ms (25000)") -> [w627]
    stop <- FALSE stop-if-true
    n370 = TCP Create Listener(10:w627) -> (0:w626:errorcluster, 3:w628:refnum<k5>)  [unwired: 4 in, 1 out]
    n371 = case shown="No Error" w626 {
      selector: w626 -> [w630 _]
      tunnel: w628 -> [w631 _]
      frame No Error {
        n372 = while {
          tunnel: w631 -> [w634]
          tunnel: w630 -> [w633]
          stop <- FALSE stop-if-true
          n373 = TCP Wait On Listener(8:w633, 11:w634) -> (0:w635:errorcluster, 4:w636:refnum<k5>)  [unwired: 2 in, 3 out]
          n374 = local write "TCP"(w636) -> ()
          n375 = case shown="No Error" w635 {
            frame No Error {
            }
            frame Error {
              n376 = Wait (ms)(milliseconds to wait=u32 1000) -> ()  [unwired: 1 out]
            }
          }
        }
      }
      frame Error {
        n377 = Wait (ms)(milliseconds to wait=u32 1000) -> ()  [unwired: 1 out]
      }
    }
  }
  n378 = local write "DB Camera Config"(w29) -> ()
  n379 = local write "Command Params"(string[][] [] ("Command Params")) -> ()
  n380 = global write "WPI_DashboardLogging Global.vi" "Recording"(w55) -> ()
  n381 = local write "Command Selection"(u16 0 ("milliseconds to wait")) -> ()
  n382 = local write "Rec Mode"(w55) -> ()
